vi "Hit Splitter.vi"(8 "error in (no error)":errorcluster, 10 "Coords":T2, 11 "Splitter in":refnum<class "Splitter.lvclass">) -> (0 "error out":errorcluster, 1 "Hit?":bool, 2 "Limits":cluster{"Left":i16, "Right":i16}, 3 "Splitter out":refnum<class "Splitter.lvclass">, 4 "Slider":T1={"Left"=0.0, "Top"=0.0, "Right"=1.0, "Bottom"=0.0}, 5 "vertical?":bool, 6 "Position":i16)   [LabVIEW 2021, in "Splitter.lvclass"]
doc: "Copyright 2018, Wiebe Walstra, wiebe@carya.nl."
uses:
  Splitter.lvclass
  C:/Projects/Dynamic-Scaling/Dynamic Scaling/IObject.lvclass
  C:/Projects/Dynamic-Scaling/Dynamic Scaling/IContainer/Divider/Divider.lvclass
  <vilib>/Utility/miscctls.llb/LVPoint32TypeDef.ctl
  Splitter.lvclass/Splitter.ctl
  Divider.lvclass
  IObject.lvclass
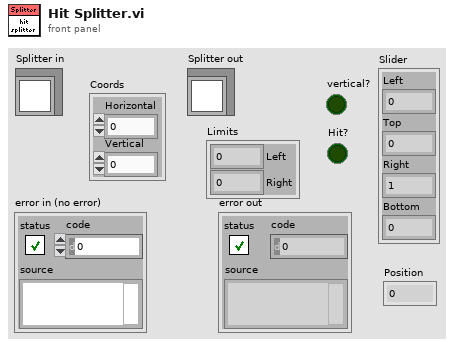
[diagram p1: front panel]
types:
  T1 = cluster{"Left":dbl, "Top":dbl, "Right":dbl, "Bottom":dbl}
  T2 = typedef "LVPoint32TypeDef.ctl" = cluster{"Horizontal":i32, "Vertical":i32}
  T3 = typedef "LVRectTypeDef.ctl" = cluster{"Left":i16, "Top":i16, "Right":i16, "Bottom":i16}
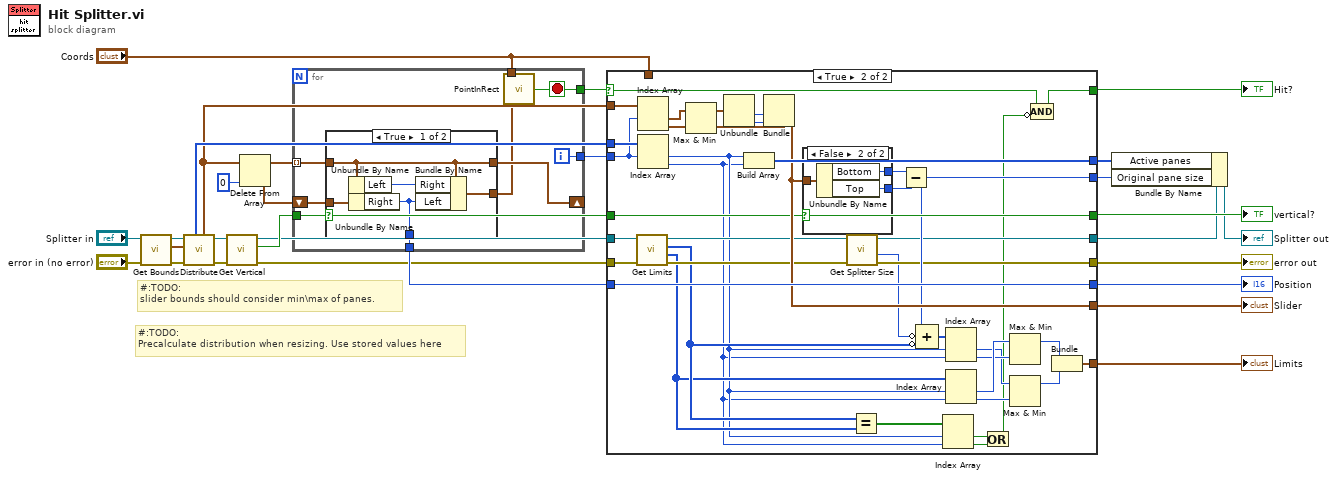
[diagram p0: block diagram]
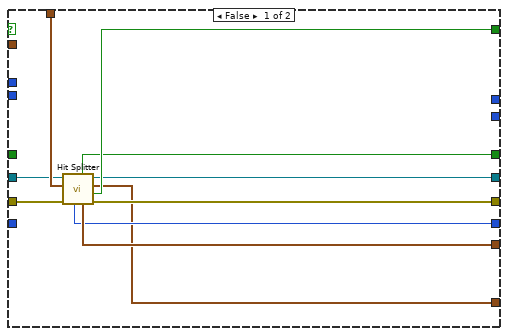
[diagram p2: hidden frame]
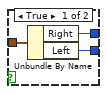
[diagram p3: hidden frame]
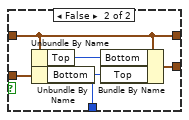
[diagram p4: hidden frame]
diagram:
  # "#:TODO:\nPrecalculate distribution when resizing. Use stored values here"
  # "#:TODO:\nslider bounds should consider min\\max of panes."
  n1 = call "Get Bounds.vi"("error in (no error)"="error in (no error)", "IObject in"="Splitter in") -> ("error out"=w27:errorcluster, "Bounds"=w14:T3, "IObject out"=w2:refnum<class "Splitter.lvclass">)  [unwired: 7 in]
  n2 = call-dynamic "Distribute.vi"("error in (no error)"=w27, "Bounds"=w14, "Container in"=w2) -> ("error out"=w26:errorcluster, "Container out"=w4:refnum<class "Splitter.lvclass">, "Visible bounds"=w8:T3[], "Visible indices"=w9:i32[])  [unwired: 4 in, 1 out]
  n3 = call "Get Vertical.vi"("error in (no error)"=w26, "Divider in"=w4) -> ("error out"=w5:errorcluster, "Vertical"=w3:bool, "Divider out"=w1:refnum<class "Splitter.lvclass">)  [unwired: 7 in]
  n4 = Delete From Array(array=w8, index=0) -> (deleted portion=w23:T3, array with subset deleted=w25:T3[])  [unwired: 1 in]
  n5 = for {
    tunnel: w25 -> [w37] mode=indexing
    shift-right: [w36] -> _
    shift-left: w23 -> [w38]
    tunnel: w3 -> [w35]
    tunnel: "Coords" -> [w34]
    tunnel: [w32] -> w19
    tunnel: [w31] -> w15
    tunnel: [w30] -> w10
    i -> [w30]
    stop <- w32 stop-if-true
    n6 = case shown="True" w35 {
      tunnel: w38 -> [w43 w48]
      tunnel: w37 -> [w42 w47]
      tunnel: [w42 w47] -> w36
      tunnel: [w41 w46] -> w33
      tunnel: [w39 w44] -> w31
      frame True {
        n7 = Unbundle By Name(w42) -> ("Left"=w40:i16)
        n8 = Unbundle By Name(w43) -> ("Right"=w39:i16)
        n9 = Bundle By Name(cluster=w42, "Right"=w40, "Left"=w39) -> (w41:T3)
      }
      frame False {
        n10 = Unbundle By Name(w47) -> ("Top"=w45:i16)
        n11 = Unbundle By Name(w48) -> ("Bottom"=w44:i16)
        n12 = Bundle By Name(cluster=w47, "Bottom"=w45, "Top"=w44) -> (w46:T3)
      }
    }
    n13 = call <vilib>:"PointInRect.vi"("rect"=w33, "point"=w34) -> ("pt in rect"=w32:bool)
  }
  n14 = case shown="True" w19 {
    selector: w19 -> [_ w61]
    tunnel: w5 -> [w51 w99]
    tunnel: w1 -> [w52 w73]
    tunnel: [w50 w70] -> w13
    tunnel: "Coords" -> [w58 _]
    tunnel: [w57 w87] -> w21
    tunnel: [w56 w72] -> w20
    tunnel: [w55 w60] -> w18
    tunnel: w3 -> [_ w86]
    tunnel: [w54 w86] -> w17
    tunnel: [w53 w88] -> w16
    tunnel: w15 -> [_ w88]
    tunnel: [_ w98] -> w11
    tunnel: w10 -> [_ w95]
    tunnel: w9 -> [_ w97]
    tunnel: w8 -> [_ w96]
    tunnel: [_ w79] -> w7
    tunnel: [w49 w80] -> w6
    frame False {
      n15 = call-parent "Hit Splitter.vi"("error in (no error)"=w51, "Point32"=w58, "IContainer in"=w52) -> ("error out"=w56:errorcluster, "Hit?"=w55:bool, "Limits"=w49:cluster{"Left":i16, "Right":i16}, "IContainer out"=w50:refnum<class "Splitter.lvclass">, "Slider"=w57:T1, "vertical?"=w54:bool, "Position"=w53:i16)  [unwired: 2 in]
    }
    frame True {
      n16 = call "Get Limits.vi"("error in (no error)"=w99, "Divider in"=w73) -> ("error out"=w74:errorcluster, "Minimal sizes"=w67:i16[], "Maximal size"=w68:i16[], "Divider out"=w71:refnum<class "Splitter.lvclass">)  [unwired: 6 in]
      n17 = Index Array(array=w96, index #1=w95) -> (element #1=w94:T3, element #2=w93:T3)  [unwired: 1 in]
      n18 = Index Array(array=w97, index #1=w95) -> (element #1=w65:i32, element #2=w64:i32)  [unwired: 1 in]
      n19 = Max & Min(x=w94, y=w93) -> (max(x,y)=w92:T3, min(x,y)=w91:T3)
      n20 = Unbundle(w92) -> ("Right"=w90:i16, "Bottom"=w89:i16)  [unwired: 2 out]
      n21 = Build Array(w65, w64) -> (w98:i32[])
      n22 = Bundle(cluster=w91, "Right"=w90, "Bottom"=w89) -> (w87:T3)  [unwired: 2 in]
      n23 = case shown="False" w86 {
        tunnel: w87 -> [w102 w105]
        tunnel: [w101 w104] -> w85
        tunnel: [w100 w103] -> w84
        frame True {
          n24 = Unbundle By Name(w102) -> ("Right"=w101:i16, "Left"=w100:i16)
        }
        frame False {
          n25 = Unbundle By Name(w105) -> ("Bottom"=w104:i16, "Top"=w103:i16)
        }
      }
      n26 = call "Get Splitter Size.vi"("error in (no error)"=w74, "Divider in"=w71) -> ("error out"=w72:errorcluster, "Splitter size"=w69:i16, "Divider out"=w70:refnum<class "Splitter.lvclass">)  [unwired: 6 in, 1 out]
      n27 = Equal?(x=w68, y=w67) -> (x = y?=w66:bool[])
      n28 = Subtract(x=w85, y=w84) -> (x-y=w79:i16)
      n29 = Compound Arithmetic op=ADD(w79, invert w69, invert w68) -> (w83:i16[])
      n30 = Index Array(array=w66, index #1=w65, index #2=w64) -> (element #1=w62:bool, element #2=w63:bool)
      n31 = Index Array(array=w83, index #1=w65, index #2=w64) -> (element #1=w76:i16, element #2=w77:i16)
      n32 = Index Array(array=w67, index #1=w65, index #2=w64) -> (element #1=w78:i16, element #2=w75:i16)
      n33 = Or(x=w62, y=w63) -> (x .or. y?=w59:bool)
      n34 = Max & Min(x=w78, y=w77) -> (max(x,y)=w82:i16)  [unwired: 1 out]
      n35 = Max & Min(x=w76, y=w75) -> (max(x,y)=w81:i16)  [unwired: 1 out]
      n36 = Compound Arithmetic op=AND(w61, invert w59) -> (w60:bool)
      n37 = Bundle(w82, w81) -> (w80:cluster{i16, i16})  [unwired: 1 in]
    }
  }
  "error out" <- w20
  "Slider" <- w21
  "Hit?" <- w18
  "vertical?" <- w17
  "Position" <- w16
  "Limits" <- w6
  n38 = Bundle By Name(cluster=w13, "Active panes"=w11, "Original pane size"=w7) -> (→"Splitter out":refnum<class "Splitter.lvclass">)
